vi "pread async serial.vi"(9 "bsize":i32, 10 "buf":i8, 11 "h":u32) -> (2 "buf out":i8, 3 "function return":i32)   [LabVIEW 2010, in "libcommon_serial.lvlib"]
doc: "int pread_async_serial(pserial_handle_t h, char*buf,int bsize);"
uses:
  <userlib>/libcommon_serial/libcommon_serial.lvlib
  <userlib>/libcommon_serial/libcommon_serial.so
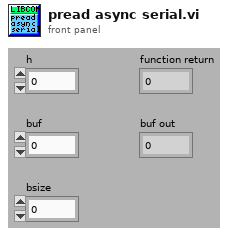
[diagram p1: front panel]
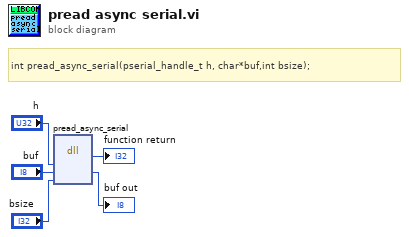
[diagram p0: block diagram]
diagram:
  # "int pread_async_serial(pserial_handle_t h, char*buf,int bsize);"
  n1 = dll-call lib="usr/local/natinst/LabVIEW-2010/user.lib/libcommon_serial/libcommon_serial.*" fn="pread_async_serial"("h"="h", "buf"="buf", "bsize"="bsize") -> (→"function return":i32, "buf"=→"buf out":i8)  [unwired: 5 in, 2 out]
